vi "Image Processing Handler Module SM.vi"(6 "Identifier":string, 8 "data queue":refnum<queue>, 9 "tx data queue":refnum<queue>, 10 "Camera? (F)":bool, 11 "Video Processor":refnum<class "Video Processor.lvclass">) -> ()   [LabVIEW 2018, in "Headless Image Processing Handler.lvclass"]
uses:
  Headless Image Processing Handler.lvclass
  <userlib>/Jet Engineering/JET_QSM/Code/Private/JET_QSM - Add State [String API].vi
  <userlib>/Jet Engineering/JET_QSM/Code/Private/JET_QSM_InvalidOption STYP.ctl
  Message/Message.lvclass
  Frame Data Message/Frame Data Message.lvclass
  ROIed Video Frame/ROIed Video Frame.lvclass
  Video Processor/Video Processor.lvclass
  Depth Data Message/Depth Data Message.lvclass
  Video Frame/Video Frame.lvclass
  C:/Users/aaron.jencks/Documents/GitHub/emerson_seed_object_detection/LabVIEW/Projects/Paul's Video Viewer/Classes/Message/Message.lvclass
  C:/Users/aaron.jencks/Documents/GitHub/emerson_seed_object_detection/LabVIEW/Projects/Paul's Video Viewer/Classes/Video Frame/Video Frame.lvclass
panel:
  out "Recent states before Error (with tick counts) 2":string="0.167 sec ago: VI Initialize\n0.167 sec ago: Window Open\n0.110 sec ago: Control Update\n0.110 sec ago: Indicator Update\n0.000 sec ago: Error Handler\r\n"
  out "error out":errorcluster
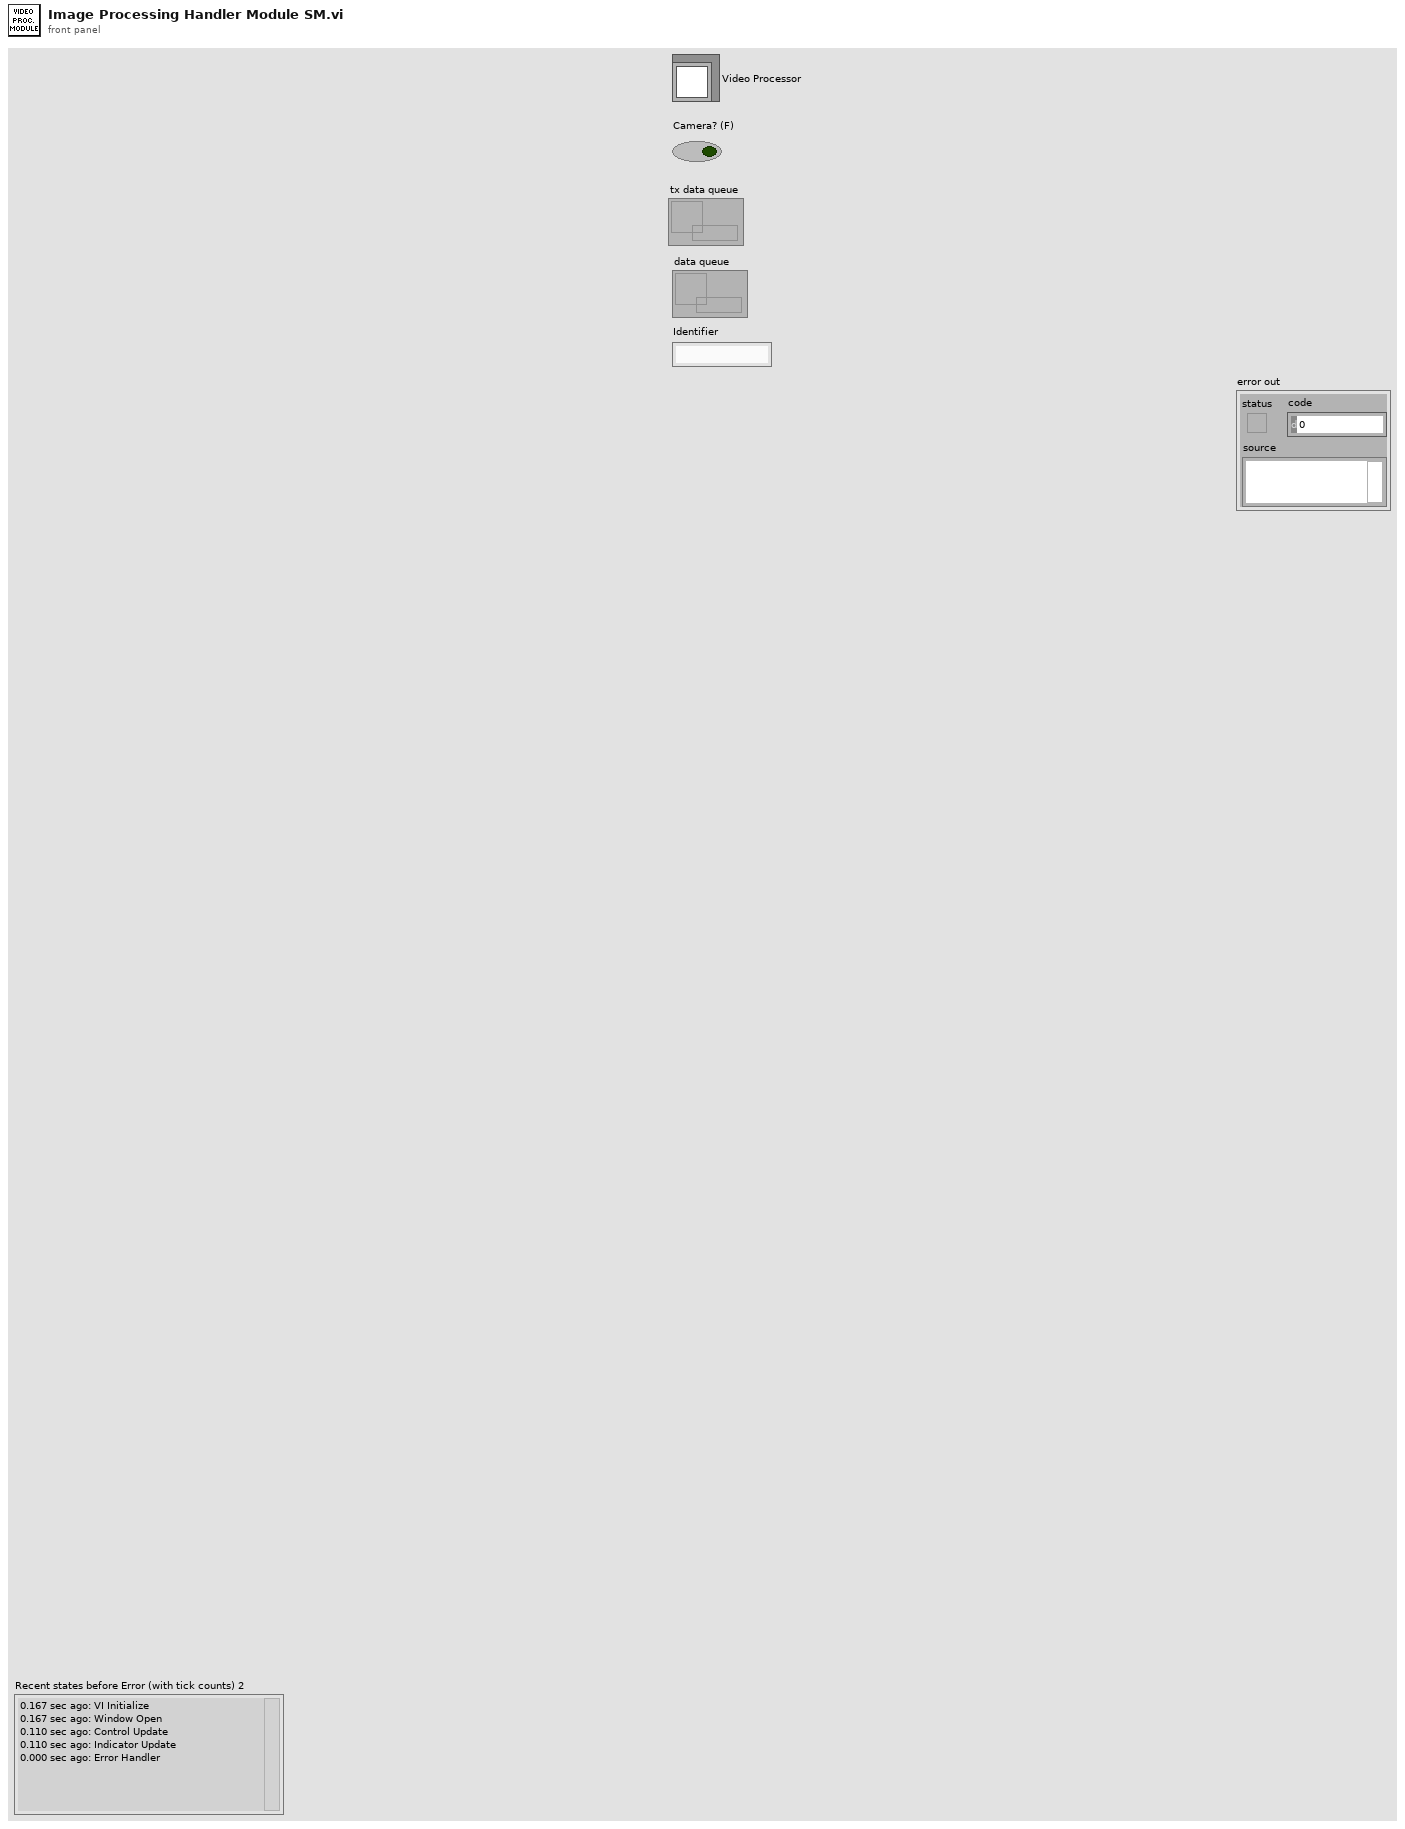
[diagram p1: front panel]
types:
  T1 = cluster{"Normal":cluster{"Averages":cluster{"Average":dbl, "RMS":dbl, "Absolute Mean Deviation":dbl}, "Global Heuristics":cluster{"Max":dbl, "Min":dbl, "Max Peak-to-Peak":dbl}, "Skewdness":dbl, "Kurtosis":dbl, "RzDIN":dbl, "RzJIS":dbl}, "Slope Parameters":cluster{"Rdq":dbl, "Rda":dbl}, "Areal Roughness":cluster{"Peak Density":dbl}}
  T2 = typedef "JET_QSM_InvalidOption STYP.ctl" = enum16{"Ignore", "Dialog", "Error"}
  T3 = typedef "JET_QSM_Refnum STYP.ctl" = cluster{"state":cluster{"queue":refnum<queue>, "idle":string, "error":string, "STOP":string}, "debug":cluster{"enabled?":bool, "queue":refnum<queue>}, "Invalid.option":T2, "QSM.Name":string}
  T4 = enum32{"invalid app kind", "Development System", "Run Time System", "Student Edition", "Embedded LabVIEW", "Evaluation", "Custom"}
  T5 = typedef "JET_QSM_Element STYP.ctl" = cluster{"state":string, "data":variant, "comment":string}
  T6 = typedef "ROI Descriptor" = cluster{"Global Rectangle":i32[], "Contours":cluster{"ID":enum32{"External", "Internal"}, "Type":u32, "Coordinates":i32[]}[]}
  T7 = cluster{"Width":u32, "Height":u32, "Frames Per Second":u32, "Codec":string, "Has Data":bool}
  T8 = typedef "IMAQ Image.ctl" = refnum<image>
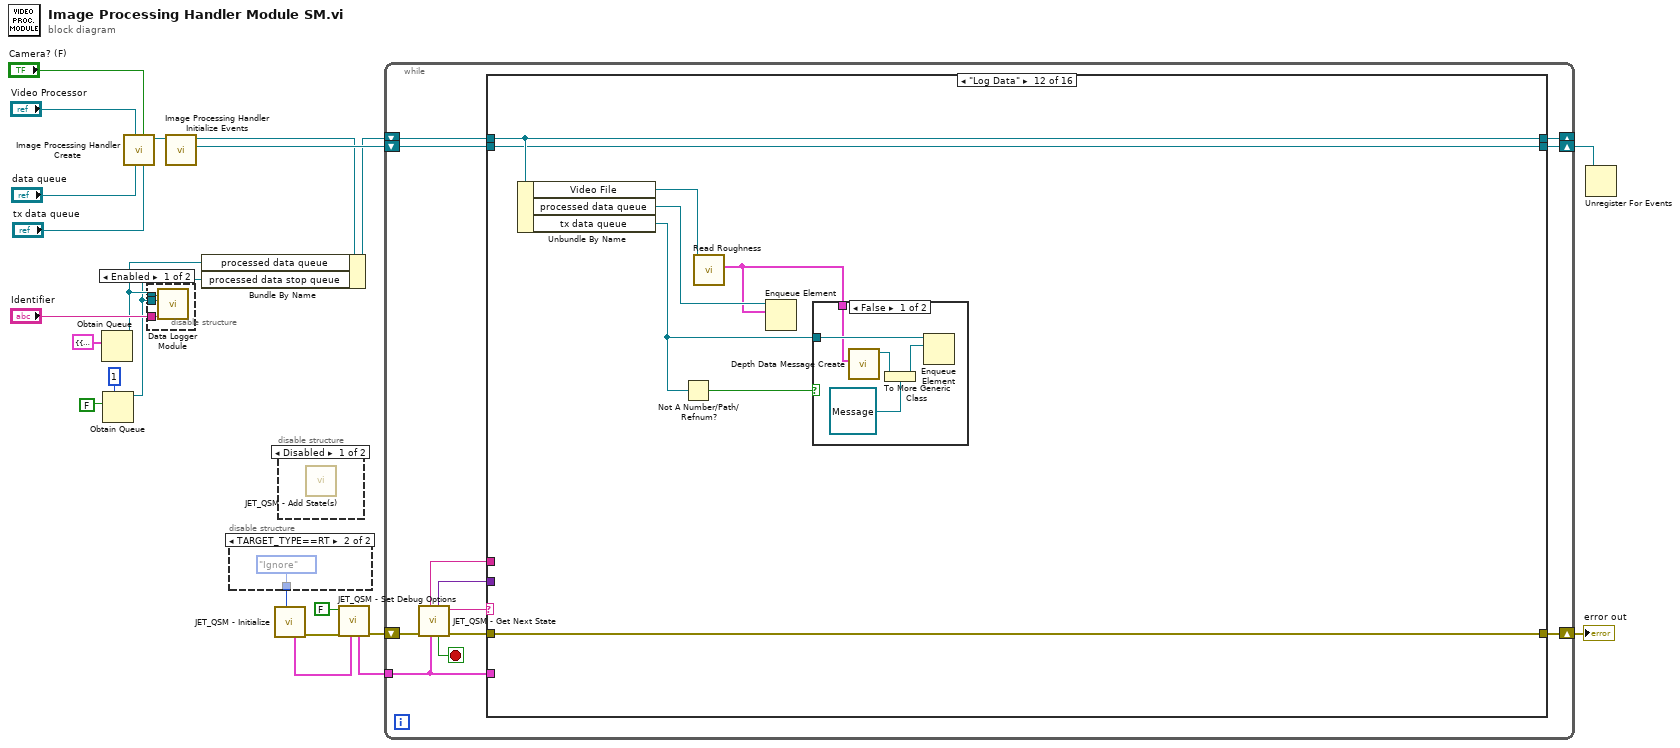
[diagram p0: block diagram]
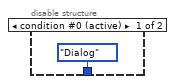
[diagram p3: hidden frame]
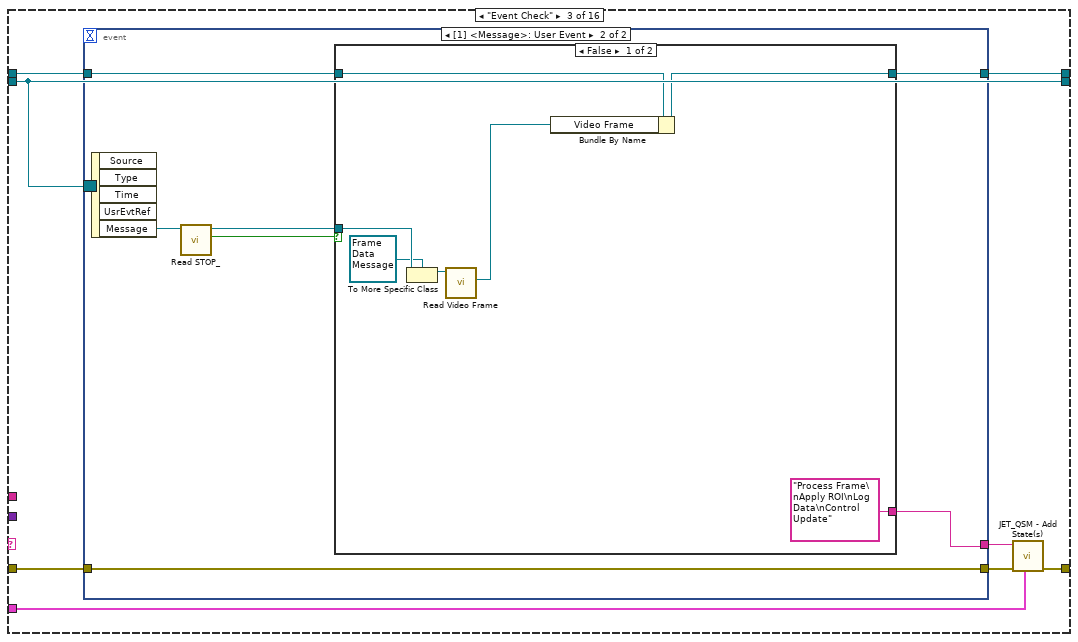
[diagram p7: hidden frame]
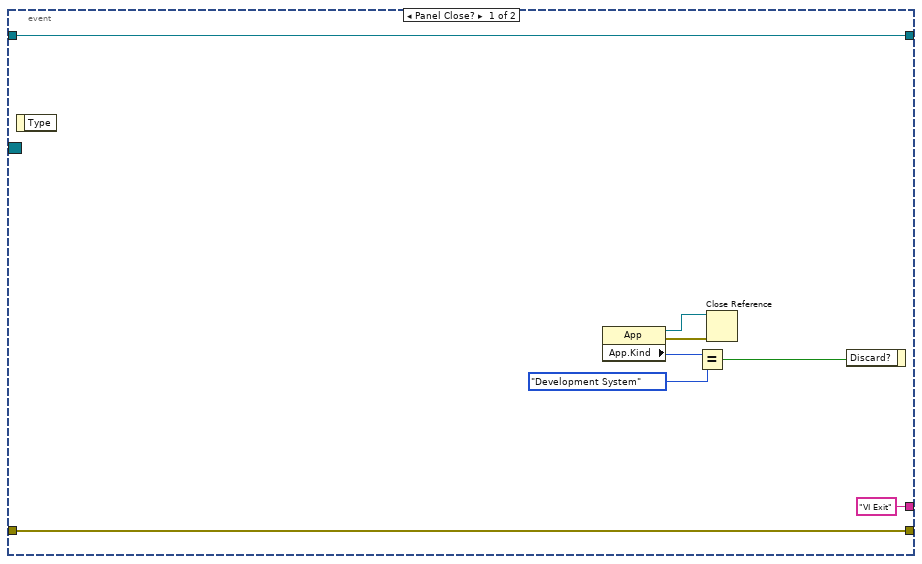
[diagram p8: hidden frame]
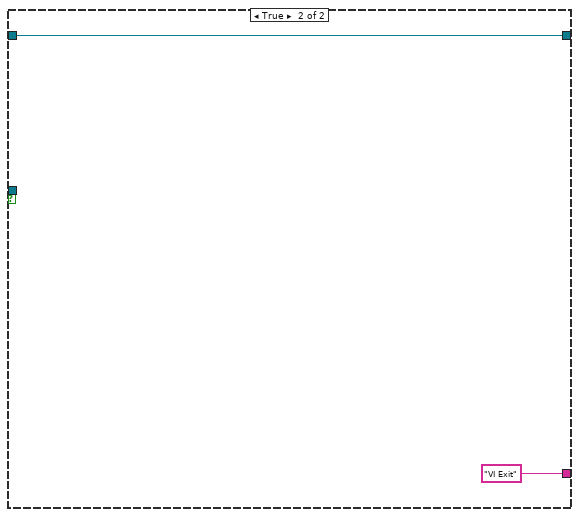
[diagram p9: hidden frame]
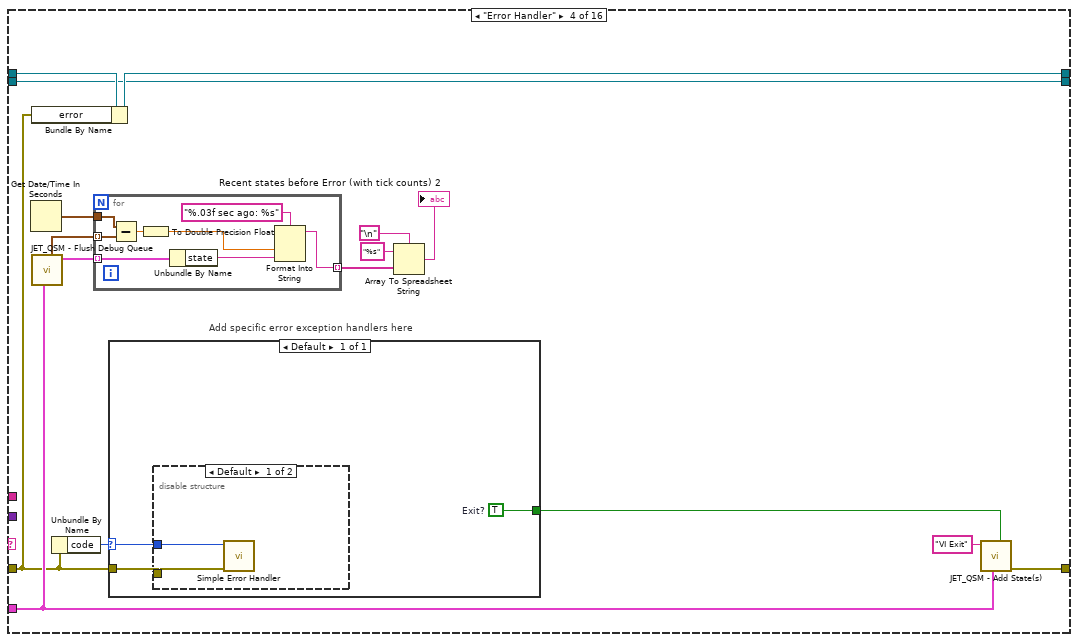
[diagram p10: hidden frame]
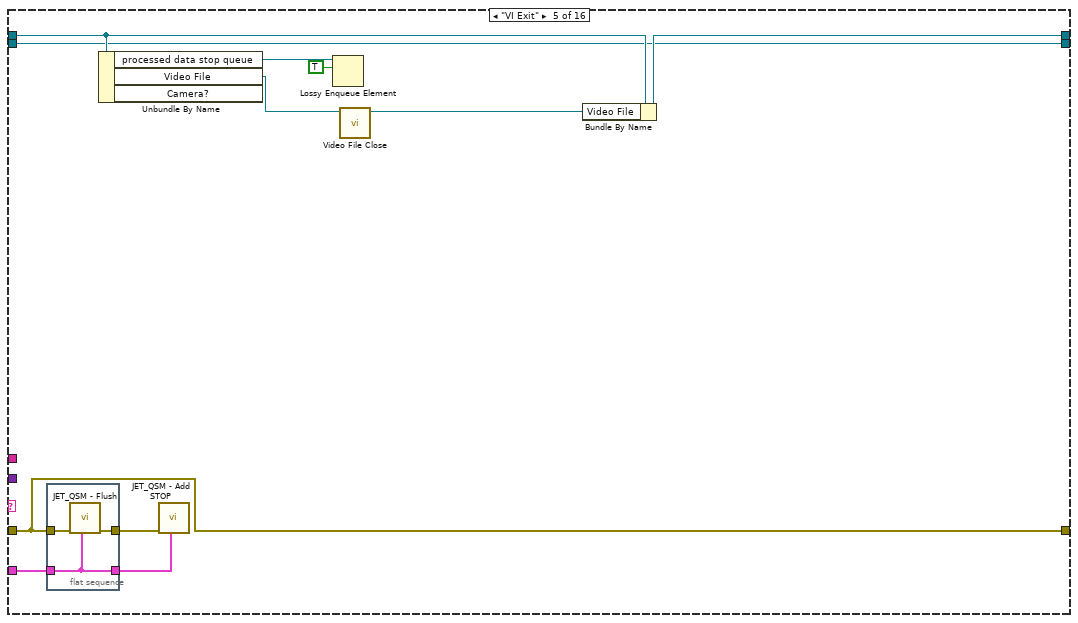
[diagram p12: hidden frame]
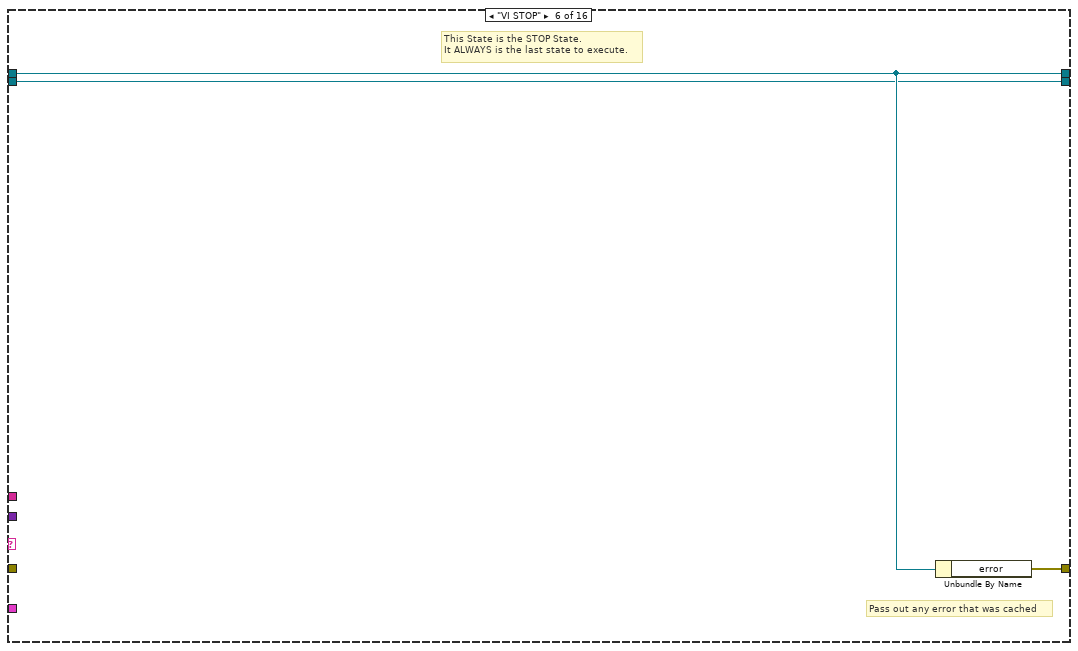
[diagram p13: hidden frame]
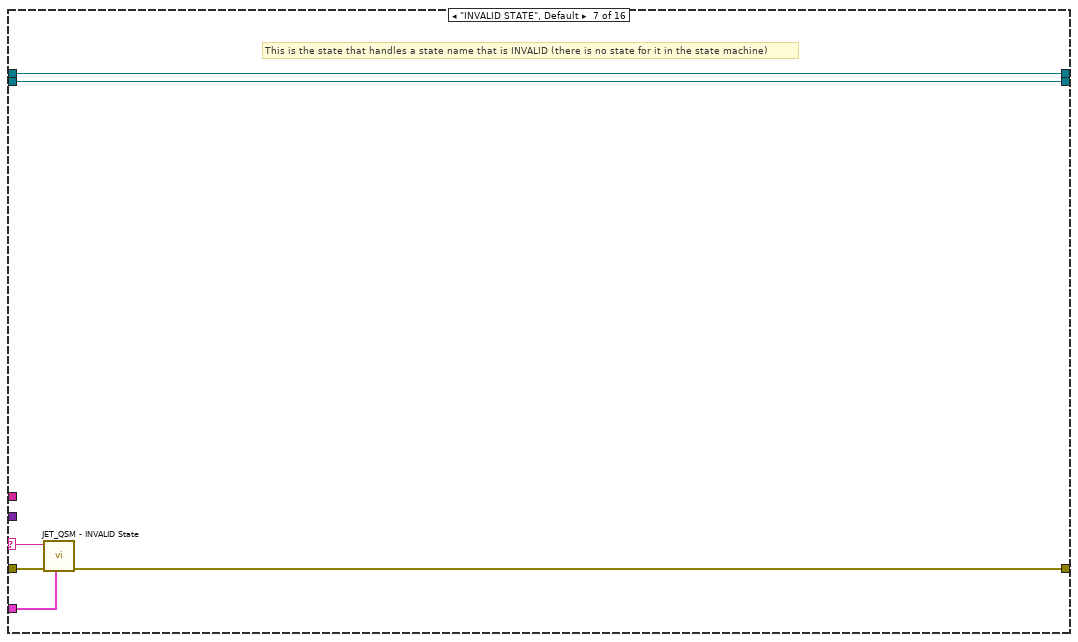
[diagram p14: hidden frame]
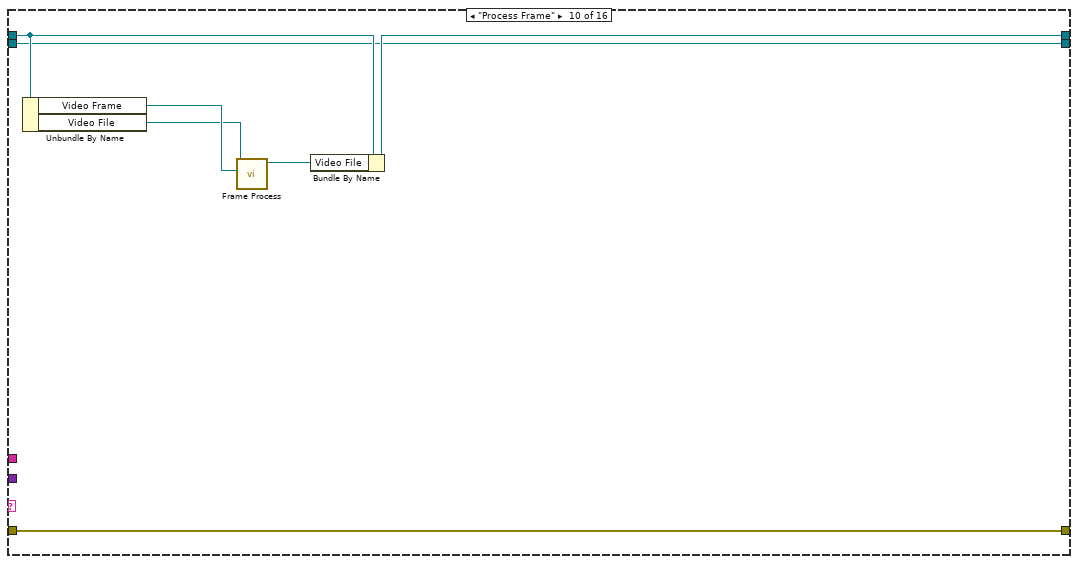
[diagram p17: hidden frame]
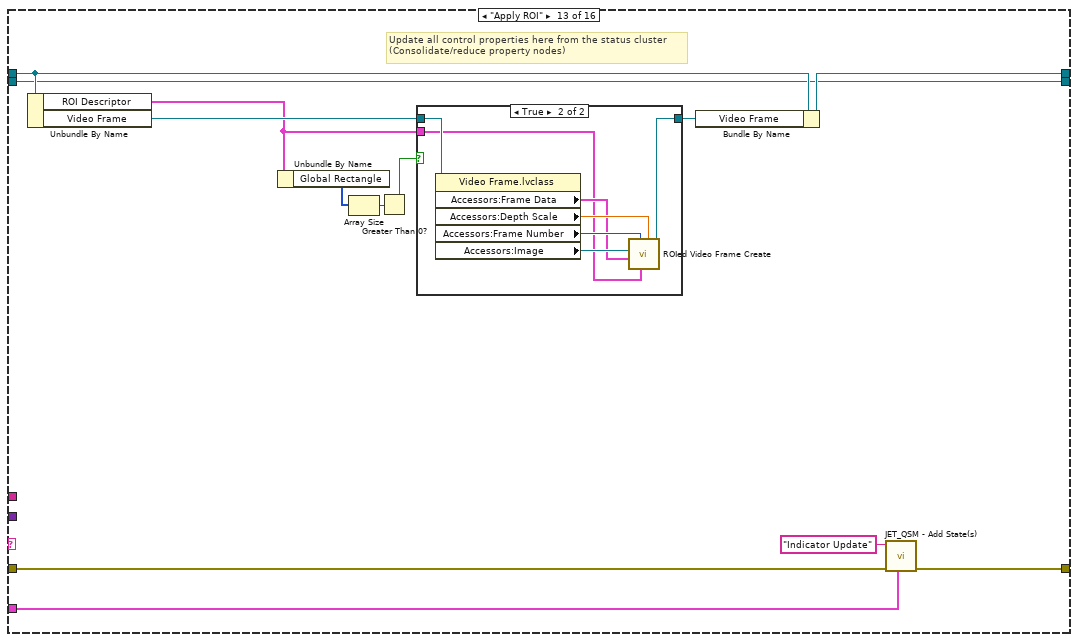
[diagram p20: hidden frame]
diagram:
  n1 = Obtain Queue(element data type=T1 {"Normal"={"Averages"={"Average"=0.0, "RMS"=0.0, "Absolute Mean Deviation"=0.0}, "Global Heuristics"={"Max"=0.0, "Min"=0.0, "Max Peak-to-Peak"=0.0}, "Skewdness"=0.0, "Kurtosis"=0.0, "RzDIN"=0.0, "RzJIS"=0.0}, "Slope Parameters"={"Rdq"=0.0, "Rda"=0.0}, "Areal Roughness"={"Peak Density"=0.0}} ("Roughness Parameters")) -> (queue out=w5:refnum<queue>)  [unwired: 4 in, 2 out]
  n2 = Obtain Queue(max queue size (-1, unlimited)=1, element data type=FALSE) -> (queue out=w4:refnum<queue>)  [unwired: 3 in, 2 out]
  n3 = call "Image Processing Handler Create.vi"("tx data queue"="tx data queue", "Camera? (F)"="Camera? (F)", "data queue"="data queue", "Video Processor"="Video Processor") -> ("Image Processing Handler out"=w15:refnum<class "Headless Image Processing Handler.lvclass">)  [unwired: 6 in, 1 out]
  n4 = disable-structure shown="Enabled" {
    disable-tunnel: "Identifier" -> [w25 _]
    disable-tunnel: w5 -> [w24 _]
    disable-tunnel: w4 -> [w23 _]
    frame Enabled {
      n5 = call "Data Logger Module.vi"("Identifier"=w25, 10:w23, "Message queue"=w24) -> ()  [unwired: 9 in]
    }
    frame Disabled {
    }
  }
  n6 = call-dynamic "Image Processing Handler Initialize Events.vi"("Image Processing Handler in"=w15) -> ("Event Registration Refnum"=w14:refnum<event-registration>, "Image Processing Handler out"=w7:refnum<class "Headless Image Processing Handler.lvclass">)  [unwired: 8 in, 1 out]
  n7 = Bundle By Name(cluster=w7, "processed data queue"=w5, "processed data stop queue"=w4) -> (w6:refnum<class "Headless Image Processing Handler.lvclass">)
  n8 = disable-structure shown="TARGET_TYPE==RT" {
    disable-tunnel: [JET_QSM_InvalidOption_STYP."Dialog" ("invalid state action (Dialog)") JET_QSM_InvalidOption_STYP."Ignore" ("invalid state action (Dialog)")] -> w22
    frame condition #0 (active) {
    }
    frame condition #1 {
    }
  }
  n9 = call <userlib>:"JET_QSM - Initialize.vi"("invalid state action (Dialog)"=w22) -> ("error out"=w16:errorcluster, "Jet_QSM refnum"=w19:T3)  [unwired: 9 in]
  n10 = disable-structure shown="Disabled" {
    frame Disabled {
      n11 = call-poly <userlib>:"JET_QSM - Add State(s).vi"() -> ()  [unwired: 11 in, 1 out]
    }
    frame Enabled {
    }
  }
  n12 = call <userlib>:"JET_QSM - Set Debug Options.vi"("Jet_QSM refnum"=w19, "error in (no error)"=w16, "debug.enabled? (F)"=FALSE) -> ("error out"=w17:errorcluster, "Jet_QSM ref"=w18:T3)  [unwired: 7 in]
  n13 = while {
    tunnel: w18 -> [w35]
    shift-right: [w33] -> _
    shift-left: w6 -> [w34]
    shift-right: [w32] -> w21
    shift-left: w17 -> [w39]
    shift-right: [w28] -> w3
    shift-left: w14 -> [w29]
    stop <- w36 stop-if-true
    n14 = call <userlib>:"JET_QSM - Get Next State.vi"("Jet_QSM refnum"=w35, "error in (no error)"=w39) -> ("error out"=w38:errorcluster, "state"=w37:string, "Stop Loop?"=w36:bool, "state data"=w31:variant, "state comment"=w30:string)  [unwired: 5 in]
    n15 = case shown="\"Log Data\"" w37 {
      selector: w37 -> [_ _ _ _ _ _ w127 _ _ _ _ _ _ _ _ _]
      tunnel: w38 -> [w41 w44 w53 w80 w117 _ w128 w131 w134 w142 w144 w153 w169 w181 w186 w190]
      tunnel: w35 -> [_ _ w52 w85 w115 _ w126 _ _ _ _ _ w170 _ w187 _]
      tunnel: w34 -> [w42 w45 w48 w81 w111 w122 w129 w132 w135 w140 w145 w152 w163 w182 w184 w191]
      tunnel: [w42 w45 w47 w79 w110 w122 w129 w132 w135 w138 w145 w152 w161 w182 w184 w191] -> w33
      tunnel: [w41 w44 w50 w86 w117 w123 w125 w131 w134 w142 w144 w153 w168 w181 w185 w190] -> w32
      tunnel: w31 -> [_ _ _ _ _ _ _ _ _ _ _ _ _ _ _ _]
      tunnel: w30 -> [_ _ _ _ _ _ _ _ _ _ _ _ _ _ _ _]
      tunnel: w29 -> [w40 w43 w46 w78 w108 w121 w124 w130 w133 w137 w143 w150 w160 w180 w183 w189]
      tunnel: [w40 w43 w46 w78 w108 w121 w124 w130 w133 w137 w143 w150 w160 w180 w183 w189] -> w28
      frame "------ Standard States ------" {
        # "Standard States are required states for a JET_QSM State Machine\n\nTheir names may be changed; use the Initialize function to specify the new names"
        # "This is a section header; the state is never expected to execute"
      }
      frame "VI Initialize" {
      }
      frame "Event Check" {
        n16 = event shown="[1] <Message>: User Event" {
          selector: w46 -> [_ _]
          dyn-events: _ -> [_ _]
          timeout: _ -> [_ _]
          tunnel: w53 -> [w55 w68]
          tunnel: ["VI Exit" ("state(s)") w65] -> w51
          tunnel: [w55 w68] -> w49
          tunnel: w48 -> [w54 w64]
          tunnel: [w54 w63] -> w47
          event Panel Close? {
            n17 = event-data() -> ()  [unwired: 1 in, 1 out]
            n18 = property class="App"() -> (reference out=w57:refnum<vi>, error out=w58:errorcluster, "App.Kind"=w61:T4)  [unwired: 2 in]
            n19 = Equal?(x=w61, y=T4."Development System") -> (x = y?=w59:bool)
            n20 = Close Reference(reference=w57, error in (no error)=w58) -> ()  [unwired: 1 out]
            n21 = event-data("Discard?"=w59) -> ()  [unwired: 1 in, 1 out]
          }
          event User Event {
            n22 = event-data() -> ("Message"=w67:refnum<class "Message.lvclass">)  [unwired: 1 in, 4 out]
            n23 = call-dynamic "Read STOP_.vi"("Message in"=w67) -> ("STOP?"=w66:bool, "Message out"=w62:refnum<class "Message.lvclass">)  [unwired: 8 in, 1 out]
            n24 = case shown="False" w66 {
              tunnel: ["Process Frame\nApply ROI\nLog Data\nControl Update" "VI Exit"] -> w65
              tunnel: w64 -> [w75 w76]
              tunnel: [w74 w76] -> w63
              tunnel: w62 -> [w73 _]
              frame False {
                n25 = To More Specific Class(target class=refnum<class "Frame Data Message.lvclass"> refnum ("Frame Data Message.lvclass"), reference=w73) -> (specific class reference=w71:refnum<class "Frame Data Message.lvclass">)  [unwired: 1 in, 1 out]
                n26 = call-dynamic "Read Video Frame.vi"("Frame Data Message in"=w71) -> ("Video Frame.lvclass"=w70:refnum<class "Video Frame.lvclass">)  [unwired: 8 in, 2 out]
                n27 = Bundle By Name(cluster=w75, "Video Frame"=w70) -> (w74:refnum<class "Headless Image Processing Handler.lvclass">)
              }
              frame True {
              }
            }
          }
        }
        n28 = call-poly <userlib>:"JET_QSM - Add State(s).vi"("Jet_QSM refnum"=w52, "error in (no error)"=w49, "state(s)"=w51) -> ("error out"=w50:errorcluster)  [unwired: 8 in]
      }
      frame "Error Handler" {
        # "Add specific error exception handlers here"
        n29 = Get Date/Time In Seconds() -> (seconds since 1Jan1904=w89:timestamp)
        n30 = Bundle By Name(cluster=w81, "error"=w80) -> (w79:refnum<class "Headless Image Processing Handler.lvclass">)
        n31 = call <userlib>:"JET_QSM - Flush Debug Queue.vi"("Jet_QSM refnum"=w85) -> ("QSM Elements"=w87:T5[], "Timestamps"=w88:timestamp[])  [unwired: 8 in, 1 out]
        n32 = Unbundle By Name(w80) -> ("code"=w82:i32)
        n33 = for {
          tunnel: w87 -> [w101] mode=indexing
          tunnel: [w99] -> w91 mode=indexing
          tunnel: w89 -> [w96]
          tunnel: w88 -> [w97] mode=indexing
          n34 = Subtract(x=w96, y=w97) -> (x-y=w95:dbl)
          n35 = To Double Precision Float(number=w95) -> (double precision float=w94:dbl)
          n36 = Unbundle By Name(w101) -> ("state"=w100:string)
          n37 = Format Into String(format string="%.03f sec ago: %s", w94, w100) -> (resulting string=w99:string)  [unwired: 2 in, 1 out]
        }
        n38 = case shown="Default" w82 {
          selector: w82 -> [w103]
          tunnel: [w104] -> w83
          tunnel: w80 -> [w102]
          frame Default {
            w104 = TRUE  # Exit?
            n39 = disable-structure shown="Default" {
              disable-tunnel: w103 -> [w106 _]
              disable-tunnel: w102 -> [w105 _]
              frame condition #0 (active) {
                n40 = call <vilib>:"Simple Error Handler.vi"("error code (no error:0)"=w106, "error in (no error)"=w105) -> ()  [unwired: 3 in, 5 out]
              }
              frame condition #1 {
              }
            }
          }
        }
        n41 = Array To Spreadsheet String(delimiter (Tab)="\n", array=w91, 3:"%s" ("format string")) -> (spreadsheet string=→"Recent states before Error (with tick counts) 2":string)
        n42 = call-poly <userlib>:"JET_QSM - Add State(s).vi"("act? (T)"=w83, "Jet_QSM refnum"=w85, "state(s)"="VI Exit") -> ("error out"=w86:errorcluster)  [unwired: 8 in]
      }
      frame "VI Exit" {
        n43 = flat-sequence {
          tunnel: w117 -> [w120]
          tunnel: [w119] -> w116
          tunnel: w115 -> [w118]
          tunnel: [w118] -> w114
          frame #0 {
            n44 = call <userlib>:"JET_QSM - Flush.vi"("Jet_QSM ref"=w118, "error in (no error)"=w120) -> ("error out"=w119:errorcluster)  [unwired: 8 in, 1 out]
          }
        }
        n45 = Unbundle By Name(w111) -> ("processed data stop queue"=w113:refnum<queue>, "Video File"=w109:refnum<class "Video Processor.lvclass">)  [unwired: 1 out]
        n46 = call <userlib>:"JET_QSM - Add STOP.vi"("Jet_QSM refnum"=w114, "error in (no error)"=w116) -> ()  [unwired: 9 in, 1 out]
        n47 = Lossy Enqueue Element(queue=w113, element=TRUE) -> ()  [unwired: 1 in, 4 out]
        n48 = call-dynamic "Video File Close.vi"("Video File in"=w109) -> ("Video File out"=w107:refnum<class "Video Processor.lvclass">)  [unwired: 9 in, 1 out]
        n49 = Bundle By Name(cluster=w111, "Video File"=w107) -> (w110:refnum<class "Headless Image Processing Handler.lvclass">)
      }
      frame "VI STOP" {
        # "Pass out any error that was cached"
        # "This State is the STOP State.\nIt ALWAYS is the last state to execute."
        n50 = Unbundle By Name(w122) -> ("error"=w123:errorcluster)
      }
      frame "INVALID STATE", Default {
        # "This is the state that handles a state name that is INVALID (there is no state for it in the state machine)"
        n51 = call <userlib>:"JET_QSM - INVALID State.vi"("Jet_QSM refnum"=w126, "error in (no error)"=w128, "state"=w127) -> ("error out"=w125:errorcluster)  [unwired: 8 in]
      }
      frame "------ Menu Commands ------" {
        # "This is a section header; the state is never expected to execute"
      }
      frame "------ Events  ------" {
        # "This is a section header; the state is never expected to execute"
      }
      frame "Process Frame" {
        n52 = Unbundle By Name(w140) -> ("Video Frame"=w141:refnum<class "Video Frame.lvclass">, "Video File"=w136:refnum<class "Video Processor.lvclass">)
        n53 = call-dynamic "Frame Process.vi"("Video Frame In"=w141, "Video Processor in"=w136) -> ("Video Processor out"=w139:refnum<class "Video Processor.lvclass">)  [unwired: 8 in, 1 out]
        n54 = Bundle By Name(cluster=w140, "Video File"=w139) -> (w138:refnum<class "Headless Image Processing Handler.lvclass">)
      }
      frame "------ Actions  ------" {
        # "This is a section header; the state is never expected to execute"
      }
      frame "Log Data" {
        n55 = Unbundle By Name(w152) -> ("Video File"=w149:refnum<class "Video Processor.lvclass">, "processed data queue"=w151:refnum<queue>, "tx data queue"=w148:refnum<queue>)
        n56 = Not A Number/Path/Refnum?(number/path/refnum=w148) -> (NaN/Path/Refnum?=w147:bool)
        n57 = call-dynamic "Read Roughness.vi"("Video Processor in"=w149) -> ("Roughness"=w146:T1)  [unwired: 8 in, 2 out]
        n58 = Enqueue Element(queue=w151, element=w146) -> ()  [unwired: 2 in, 3 out]
        n59 = case shown="False" w147 {
          tunnel: w148 -> [w158 _]
          tunnel: w146 -> [w157 _]
          frame False {
            n60 = call "Depth Data Message Create.vi"("Roughness"=w157) -> ("Depth Data Message out"=w156:refnum<class "Depth Data Message.lvclass">)  [unwired: 9 in, 1 out]
            n61 = To More Generic Class(target class=refnum<class "Message.lvclass"> refnum ("Message.lvclass"), reference=w156) -> (generic class reference=w155:refnum<class "Message.lvclass">)
            n62 = Enqueue Element(queue=w158, element=w155) -> ()  [unwired: 2 in, 3 out]
          }
          frame True {
          }
        }
      }
      frame "Apply ROI" {
        # "Update all control properties here from the status cluster\n(Consolidate/reduce property nodes)"
        n63 = Unbundle By Name(w163) -> ("ROI Descriptor"=w159:T6, "Video Frame"=w167:refnum<class "Video Frame.lvclass">)
        n64 = Unbundle By Name(w159) -> ("Global Rectangle"=w166:i32[])
        n65 = Array Size(array=w166) -> (size(s)=w165:i32)
        n66 = Greater Than 0?(x=w165) -> (x > 0?=w164:bool)
        n67 = case shown="True" w164 {
          tunnel: w167 -> [w172 w179]
          tunnel: w159 -> [_ w174]
          tunnel: [w172 w173] -> w162
          frame False {
          }
          frame True {
            n68 = property class="Video Frame.lvclass"(reference=w179) -> ("Accessors:Frame Data"=w175:T7, "Accessors:Depth Scale"=w178:dbl, "Accessors:Frame Number"=w177:i32, "Accessors:Image"=w176:T8)  [unwired: 1 in, 2 out]
            n69 = call "ROIed Video Frame Create.vi"("Depth Scale"=w178, "ROI Descriptor"=w174, "Frame Number"=w177, "Frame Data"=w175, "Image Dst"=w176) -> ("ROIed Video Frame out"=w173:refnum<class "ROIed Video Frame.lvclass">)  [unwired: 5 in, 1 out]
          }
        }
        n70 = Bundle By Name(cluster=w163, "Video Frame"=w162) -> (w161:refnum<class "Headless Image Processing Handler.lvclass">)
        n71 = call-poly <userlib>:"JET_QSM - Add State(s).vi"("Jet_QSM refnum"=w170, "error in (no error)"=w169, "state(s)"="Indicator Update") -> ("error out"=w168:errorcluster)  [unwired: 8 in]
      }
      frame "------ Window and Panel Control ------" {
        # "This is a section header; the state is never expected to execute"
      }
      frame "Control Update" {
        # "Update all control properties here from the status cluster\n(Consolidate/reduce property nodes)"
        n72 = call-poly <userlib>:"JET_QSM - Add State(s).vi"("Jet_QSM refnum"=w187, "error in (no error)"=w186, "state(s)"="Indicator Update") -> ("error out"=w185:errorcluster)  [unwired: 8 in]
      }
      frame "Indicator Update" {
        # "Update all indicator values here from the status cluster\n(Eliminate Local Variables)"
      }
    }
  }
  "error out" <- w21
  n73 = Unregister For Events(event registration refnum=w3) -> ()  [unwired: 1 in, 1 out]
